vi "Backup Data File.vi"(8 "error in (no error)":errorcluster, 10 "Back up data file?":bool, 11 "file path (use dialog)":path=path "G:/My Drive/WPC Stat Scrape/Data/WPC Stats.bin") -> (0 "error out":errorcluster)   [LabVIEW 2021]
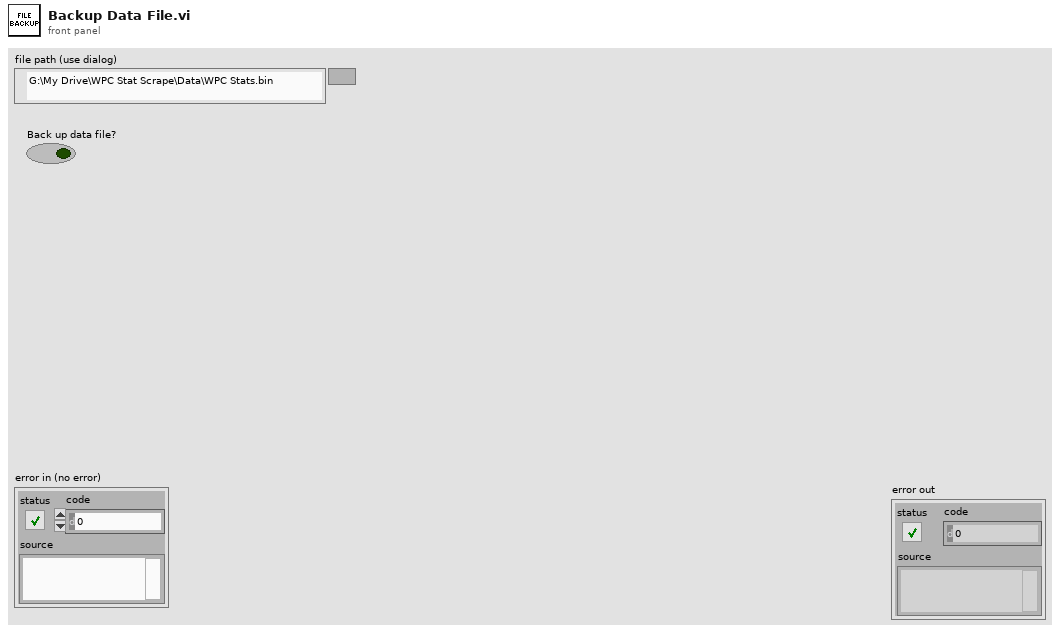
[diagram p1: front panel]
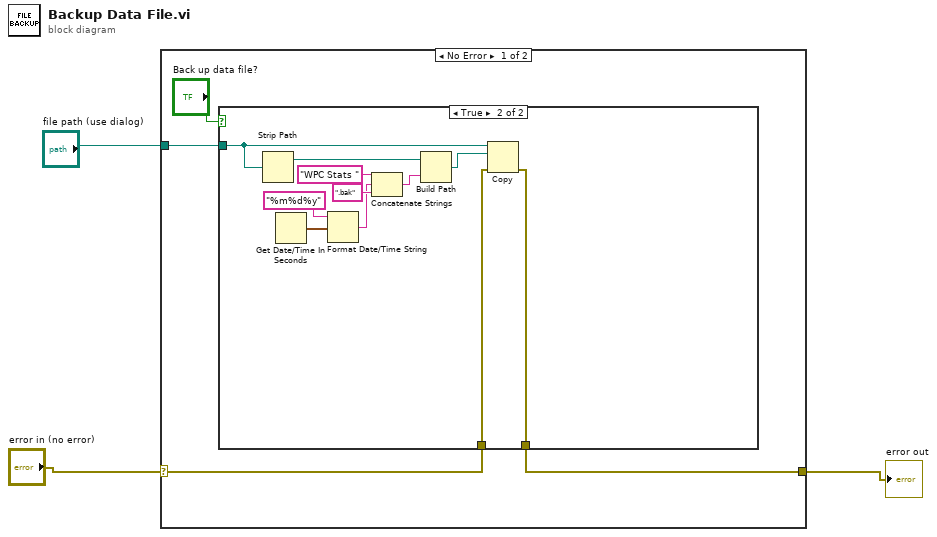
[diagram p0: block diagram]
diagram:
  n1 = case shown="No Error" "error in (no error)" {
    selector: "error in (no error)" -> [w5 w20]
    tunnel: [w4 w20] -> w2
    tunnel: "file path (use dialog)" -> [w6 _]
    frame No Error {
      n2 = case shown="True" "Back up data file?" {
        tunnel: w6 -> [_ w12]
        tunnel: w5 -> [w8 w10]
        tunnel: [w8 w9] -> w4
        frame False {
        }
        frame True {
          n3 = Strip Path(path=w12) -> (stripped path=w19:path)  [unwired: 1 out]
          n4 = Get Date/Time In Seconds() -> (seconds since 1Jan1904=w14:timestamp)
          n5 = Format Date/Time String(time format string (%c)="%m%d%y", seconds (now)=w14) -> (date/time string=w16:string)  [unwired: 1 in]
          n6 = Concatenate Strings("WPC Stats " ("string"), w16, ".bak" ("string")) -> (w13:string)
          n7 = Build Path(base path=w19, name or relative path=w13) -> (appended path=w11:path)
          n8 = Copy(8:w10, 10:w11, 11:w12) -> (0:w9:errorcluster)  [unwired: 2 in, 2 out]
        }
      }
    }
    frame Error {
    }
  }
  "error out" <- w2
